vi "Get Comparison String.vi"(8 "error in (no error)":errorcluster, 10 "Assert Message":T1, 11 "Assert Name Filter in":refnum<class "Assert Name Filter.lvclass">) -> (0 "error out":errorcluster, 2 "Comparison String":string)   [LabVIEW 2017, in "Assert API Components.lvlib" / "Assert Name Filter.lvclass"]
uses:
  Assert Name Filter.lvclass
  Message Data.ctl
  Failure Actions.ctl
  Assert API Components.lvlib
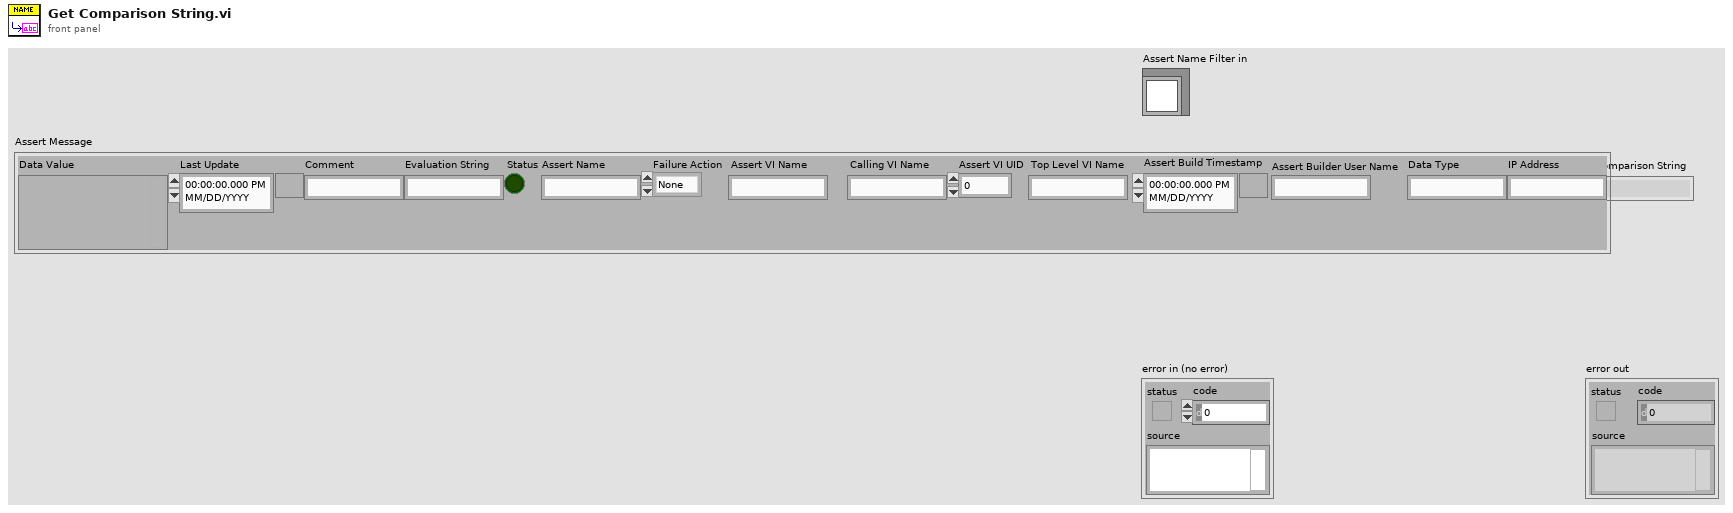
[diagram p1: front panel]
types:
  T1 = typedef "Assert API Components.lvlib/Message Data.ctl" = cluster{"Data Value":variant, "Last Update":timestamp, "Comment":string, "Evaluation String":string, "Status":bool, "Assert Name":string, "Failure Action":T2, "Assert VI Name":string, "Calling VI Name":string, "Assert VI UID":i32, "Top Level VI Name":string, "Assert Build Timestamp":timestamp, "Assert Builder User Name":string, "Data Type":string, "IP Address":string}
  T2 = typedef "Assert API Components.lvlib/Failure Actions.ctl" = enum16{"None", "Log To File", "Pause Execution", "Abort Execution"}
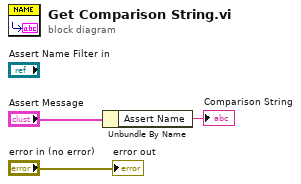
[diagram p0: block diagram]
diagram:
  n1 = Unbundle By Name("Assert Message") -> ("Assert Name"=→"Comparison String":string)
  "error out" <- "error in (no error)"
